vi "SMUVoltage.vi"() -> ()   [LabVIEW 2020]
uses:
  <instrlib>/niDCPower/nidcpower.llb/niDCPower Output Function.ctl
panel:
  out "current measurements":dbl[](array[numeric])
  out "voltage measurements":dbl[](array[numeric])
  in  "instrument handle":refnum<k15>="NI_SMU1"
  in  "error in (no error)":errorcluster
  out "error out":errorcluster
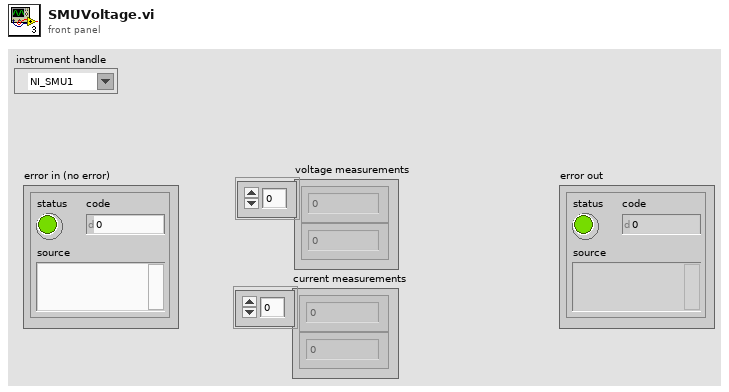
[diagram p1: front panel]
types:
  T1 = typedef "niDCPower Output Function.ctl" = i32
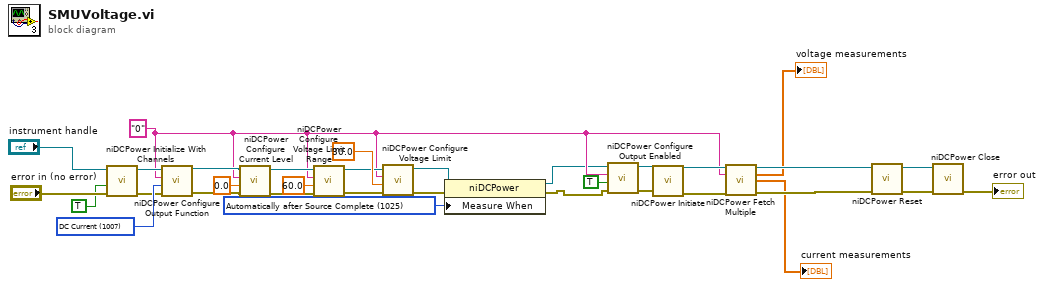
[diagram p0: block diagram]
diagram:
  w1 = 1025 items=["Automatically after Source Complete"=1025, "On Demand"=1026, "On Measure Trigger"=1027] ("Measurement:Advanced:Measure When")
  w9 = "0" ("channel name")
  w29 = T1 1007 items=["DC Voltage"=1006, "DC Current"=1007, "Pulse Voltage"=1049, "Pulse Current"=1050] ("output function")
  n1 = call <instrlib>:"niDCPower Initialize With Channels.vi"("error in (no error)"="error in (no error)", "reset (false)"=TRUE, "resource name"="instrument handle") -> ("error out"=w28:errorcluster, "instrument handle out"=w30:refnum<k15>)  [unwired: 7 in]
  n2 = call <instrlib>:"niDCPower Configure Output Function.vi"("error in (no error)"=w28, "output function"=w29, "channel name"=w9, "instrument handle"=w30) -> ("error out"=w26:errorcluster, "instrument handle out"=w27:refnum<k15>)  [unwired: 6 in]
  n3 = call <instrlib>:"niDCPower Configure Current Level.vi"("error in (no error)"=w26, "current level"=0.0, "channel name"=w9, "instrument handle"=w27) -> ("error out"=w19:errorcluster, "instrument handle out"=w18:refnum<k15>)  [unwired: 6 in]
  n4 = call <instrlib>:"niDCPower Configure Voltage Limit Range.vi"("error in (no error)"=w19, "voltage limit range"=60.0, "channel name"=w9, "instrument handle"=w18) -> ("error out"=w16:errorcluster, "instrument handle out"=w17:refnum<k15>)  [unwired: 6 in]
  n5 = call <instrlib>:"niDCPower Configure Voltage Limit.vi"("error in (no error)"=w16, "voltage limit"=30.0, "channel name"=w9, "instrument handle"=w17) -> ("error out"=w5:errorcluster, "instrument handle out"=w3:refnum<k15>)  [unwired: 6 in]
  n6 = property class="niDCPower"(reference=w3, error in=w5, "Measure When"=w1) -> (reference out=w2:refnum<k15>, error out=w4:errorcluster)
  n7 = call <instrlib>:"niDCPower Configure Output Enabled.vi"("error in (no error)"=w4, "output enabled"=TRUE, "channel name"=w9, "instrument handle"=w2) -> ("error out"=w12:errorcluster, "instrument handle out"=w11:refnum<k15>)  [unwired: 6 in]
  n8 = call <instrlib>:"niDCPower Initiate.vi"("error in (no error)"=w12, "instrument handle"=w11) -> ("error out"=w21:errorcluster, "instrument handle out"=w20:refnum<k15>)  [unwired: 2 in, 6 out]
  n9 = call <instrlib>:"niDCPower Fetch Multiple.vi"("instrument handle"=w20, "channel name"=w9, "error in (no error)"=w21) -> ("instrument handle out"=w13:refnum<k15>, "voltage measurements"=→"voltage measurements":dbl[], "current measurements"=→"current measurements":dbl[], "error out"=w14:errorcluster)  [unwired: 7 in, 2 out]
  n10 = call <instrlib>:"niDCPower Reset.vi"("error in (no error)"=w14, "instrument handle"=w13) -> ("error out"=w24:errorcluster, "instrument handle out"=w23:refnum<k15>)  [unwired: 8 in]
  n11 = call <instrlib>:"niDCPower Close.vi"("error in (no error)"=w24, "instrument handle"=w23) -> ("error out"=→"error out":errorcluster)  [unwired: 9 in]
